vi "2283_gyroPID.vi"(0 "Y Axis Input":dbl, 1 "Y Input?":bool, 2 "Angulo Actual":dbl format="%#_13g", 3 "Angulo Deseado":dbl format="%#_13g") -> (5 "Y Axis Output":dbl(slide) scale=-0.8..0.8)   [LabVIEW 2015]
uses:
  <vilib>/addons/control/pid/pid.llb/PID (DBL).vi
  <vilib>/addons/control/pid/NI_PID_pid.lvlib
panel:
  in  "PID gains":T1={"proportional gain (Kc)"=1.0, "integral time (Ti, min)"=0.01, "derivative time (Td, min)"=0.0} {"derivative time (Td, min)" format="%.3f"; "integral time (Ti, min)" format="%.3f"; "proportional gain (Kc)" format="%.3f"}
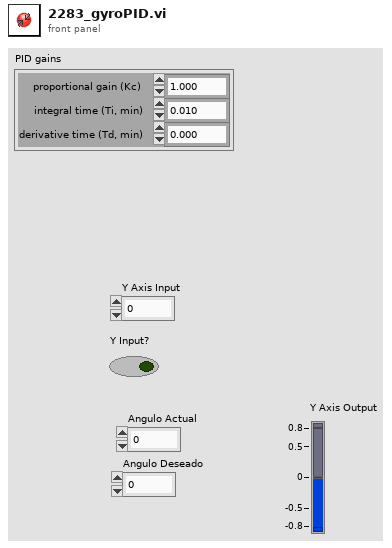
[diagram p1: front panel]
types:
  T1 = cluster{"proportional gain (Kc)":dbl, "integral time (Ti, min)":dbl, "derivative time (Td, min)":dbl}
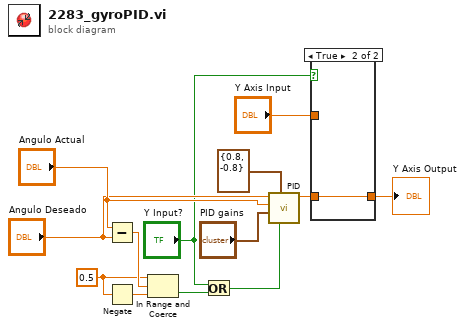
[diagram p0: block diagram]
diagram:
  w4 = 0.5
  n1 = Subtract(x="Angulo Actual", y="Angulo Deseado") -> (x-y=w8:dbl)
  n2 = Negate(x=w4) -> (-x=w5:dbl)
  n3 = In Range and Coerce(upper limit=w4, x=w8, lower limit=w5) -> (In Range?=w2:bool)  [unwired: 1 out]
  n4 = Or(x="Y Input?", y=w2) -> (x .or. y?=w3:bool)
  n5 = call-poly <vilib>:"PID.vi"("reinitialize? (F)"=w3, "output range"=cluster{"output high":dbl, "output low":dbl} {"output high"=0.8, "output low"=-0.8}, "PID gains"="PID gains", "process variable"="Angulo Actual", "setpoint"="Angulo Deseado") -> ("output"=w10:dbl)  [unwired: 5 in, 1 out]
  n6 = case shown="True" "Y Input?" {
    tunnel: [w14 w15] -> w12
    tunnel: w10 -> [_ w15]
    tunnel: "Y Axis Input" -> [w14 _]
    frame False {
    }
    frame True {
    }
  }
  "Y Axis Output" <- w12
